vi "Read Age.vi"(8 "error in (no error)":errorcluster, 11 "myClass in":refnum<class "myClass.lvclass">) -> (0 "error out":errorcluster, 2 "Age":i32, 3 "myClass out":refnum<class "myClass.lvclass">)   [LabVIEW 2012, in "myClass.lvclass"]
uses:
  myClass.lvclass
  myClass.lvclass/myClass.ctl
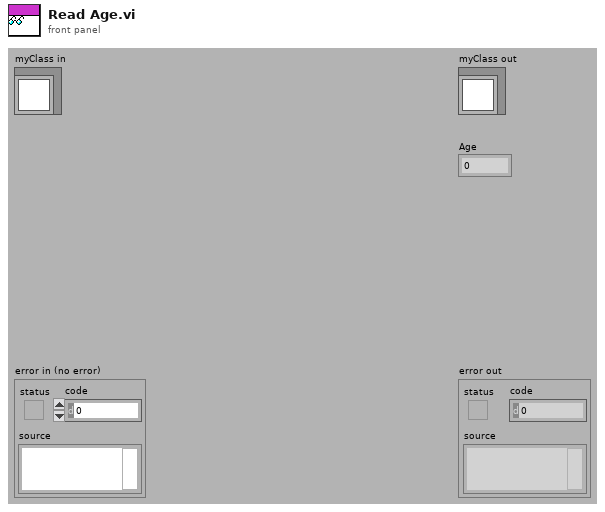
[diagram p1: front panel]
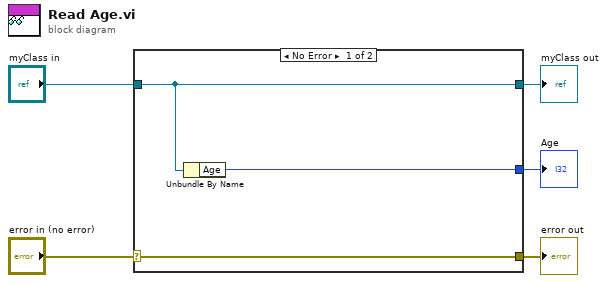
[diagram p0: block diagram]
diagram:
  n1 = case shown="No Error" "error in (no error)" {
    selector: "error in (no error)" -> [w8 w9]
    tunnel: [w8 w9] -> w4
    tunnel: [w7 w10] -> w2
    tunnel: "myClass in" -> [w7 w10]
    tunnel: [w6 _] -> w1
    frame No Error {
      n2 = Unbundle By Name(w7) -> ("Age"=w6:i32)
    }
    frame Error {
    }
  }
  "error out" <- w4
  "myClass out" <- w2
  "Age" <- w1
